vi "InstrumentErrorHandlerDialog.vi"(8 "error in (no error)":errorcluster, 11 "Select Spectrometer":refnum<visa-resource-name>="USB650") -> (0 "error out":errorcluster, 2 "Enter Viewer Mode Out":bool, 3 "Spectrometer Out":refnum<visa-resource-name>="USB650", 4 "Add Entry Pressed?":bool=TRUE)   [LabVIEW 2013]
doc: "Use this template to build a VI to use as a subVI."
panel:
  in  "Enter Viewer Mode":bool
  in  "Cancel Button":bool
  in  "Add Entry Button":bool
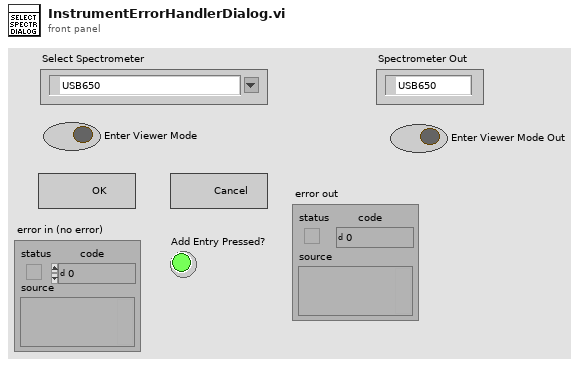
[diagram p1: front panel]
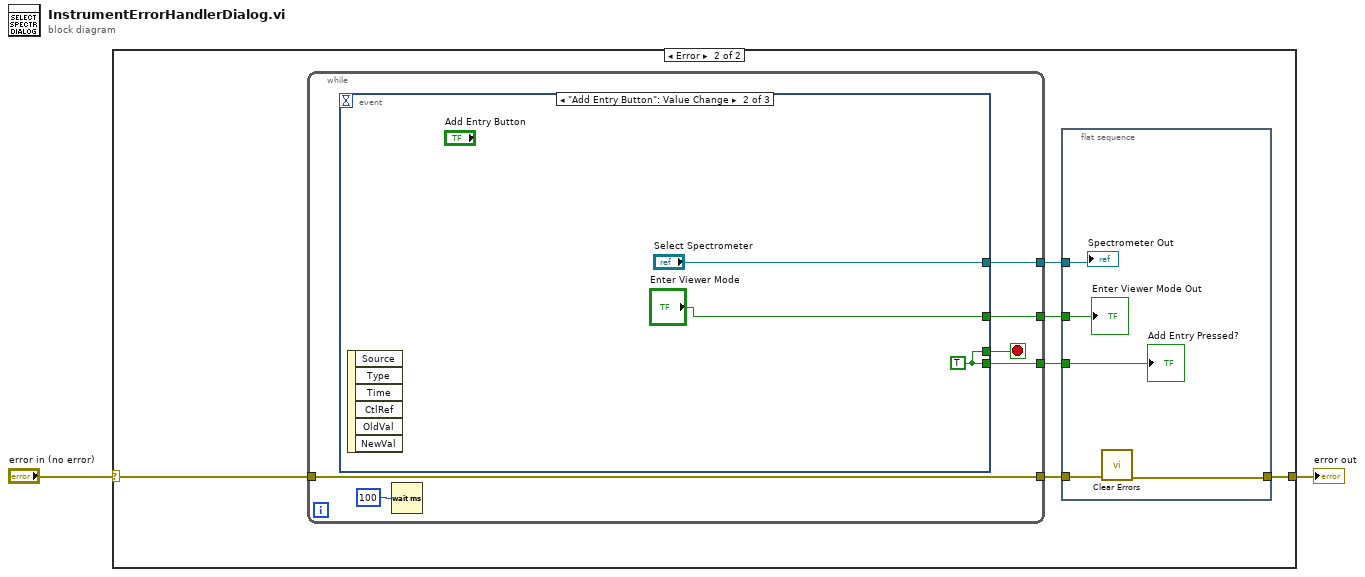
[diagram p0: block diagram]
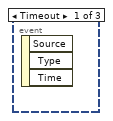
[diagram p3: hidden frame]
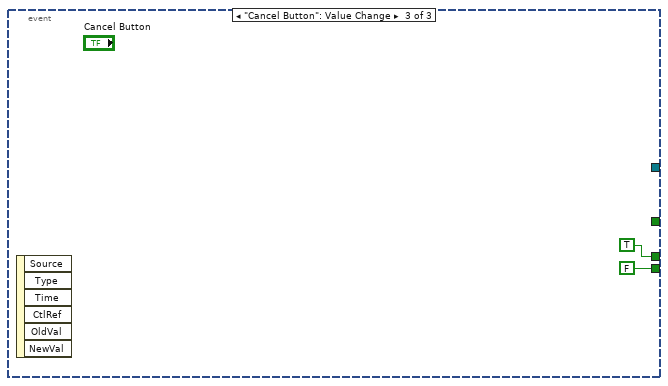
[diagram p4: hidden frame]
diagram:
  n1 = case shown="Error" "error in (no error)" {
    selector: "error in (no error)" -> [w3 w5]
    tunnel: [w3 w8] -> w1
    frame No Error {
    }
    frame Error {
      n2 = while {
        tunnel: [w19] -> w9
        tunnel: w5 -> [w17]
        tunnel: [w17] -> w7
        tunnel: [w16] -> w6
        tunnel: [w15] -> w4
        stop <- w20 stop-if-true
        n3 = event shown="[1] \"Add Entry Button\": Value Change" {
          selector: _ -> [_ _ _]
          dyn-events: _ -> [_ _ _]
          timeout: _ -> [_ _ _]
          tunnel: [_ w23 TRUE] -> w20
          tunnel: [_ w23 FALSE] -> w19
          tunnel: [_ "Select Spectrometer" _] -> w16
          tunnel: [_ "Enter Viewer Mode" _] -> w15
          event Timeout {
            n4 = event-data() -> ()  [unwired: 1 in, 3 out]
          }
          event "Add Entry Button": Value Change {
            w23 = TRUE
            n5 = event-data() -> ()  [unwired: 1 in, 6 out]
          }
          event "Cancel Button": Value Change {
            n6 = event-data() -> ()  [unwired: 1 in, 6 out]
          }
        }
        n7 = Wait (ms)(milliseconds to wait=u32 100) -> ()  [unwired: 1 out]
      }
      n8 = flat-sequence {
        tunnel: w9 -> [w14]
        tunnel: w7 -> [w12]
        tunnel: [w11] -> w8
        tunnel: w6 -> [w13]
        tunnel: w4 -> [w10]
        frame #0 {
          n9 = call <vilib>:"Clear Errors.vi"("error in (no error)"=w12) -> ("error out"=w11:errorcluster)  [unwired: 6 in]
          "Add Entry Pressed?" <- w14
          "Spectrometer Out" <- w13
          "Enter Viewer Mode Out" <- w10
        }
      }
    }
  }
  "error out" <- w1
